vi "Threshold Obstacles.vi"(8 "error in (no error)":errorcluster, 10 "Threshold":dbl, 11 "Simulator in":refnum<class "Simulator.lvclass">) -> (0 "error out":errorcluster, 2 "Obstacles Within Threshold":cluster{"x":dbl, "y":dbl}[](array[cluster]), 3 "Simulator out":refnum<class "Simulator.lvclass">)   [LabVIEW 2011, in "Simulator.lvclass"]
uses:
  Simulator.lvclass
  Simulator.lvclass/Simulator.ctl
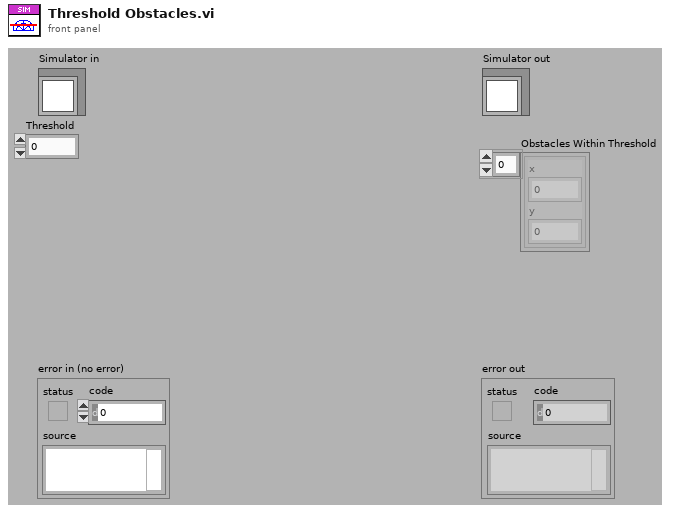
[diagram p1: front panel]
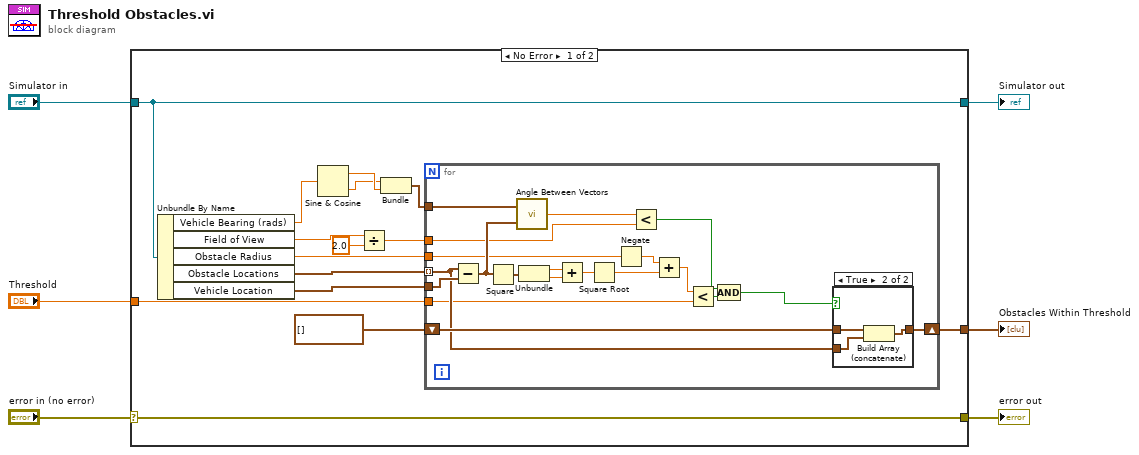
[diagram p0: block diagram]
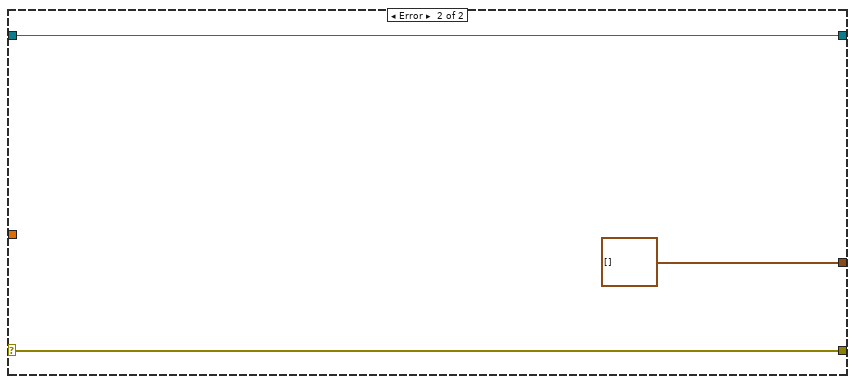
[diagram p3: hidden frame]
diagram:
  n1 = case shown="No Error" "error in (no error)" {
    selector: "error in (no error)" -> [w21 w48]
    tunnel: [w21 w48] -> w5
    tunnel: [w20 w47] -> w3
    tunnel: "Simulator in" -> [w20 w47]
    tunnel: "Threshold" -> [w16 _]
    tunnel: [w15 cluster{"x":dbl, "y":dbl}[] [] ("Obstacle Locations")] -> w1
    frame No Error {
      n2 = Unbundle By Name(w20) -> ("Vehicle Bearing (rads)"=w11:dbl, "Field of View"=w14:dbl, "Obstacle Radius"=w7:dbl, "Obstacle Locations"=w18:cluster{"x":dbl, "y":dbl}[], "Vehicle Location"=w19:cluster{"x":dbl, "y":dbl})
      n3 = Sine & Cosine(0:w11) -> (1:w9:dbl, 2:w8:dbl)
      n4 = Divide(x=w14, y=2.0) -> (x/y=w12:dbl)
      n5 = Bundle(w8, w9) -> (w10:cluster{dbl, dbl})  [unwired: 1 in]
      n6 = for {
        tunnel: w19 -> [w41]
        tunnel: w18 -> [w35] mode=indexing
        shift-right: [w34] -> w15
        shift-left: cluster{"x":dbl, "y":dbl}[] [] ("Obstacle Locations") -> [w36]
        tunnel: w16 -> [w33]
        tunnel: w12 -> [w29]
        tunnel: w10 -> [w27]
        tunnel: w7 -> [w24]
        n7 = Subtract(x=w35, y=w41) -> (x-y=w30:cluster{"x":dbl, "y":dbl})
        n8 = Square(x=w30) -> (x^2=w40:cluster{"x":dbl, "y":dbl})
        n9 = call "Angle Between Vectors.vi"("B"=w30, "A"=w27) -> ("Angle (rads)"=w28:dbl)
        n10 = Unbundle(w40) -> ("x"=w39:dbl, "y"=w38:dbl)
        n11 = Add(x=w39, y=w38) -> (x+y=w37:dbl)
        n12 = Square Root(x=w37) -> (sqrt(x)=w26:dbl)
        n13 = Negate(x=w24) -> (-x=w23:dbl)
        n14 = Less?(x=w28, y=w29) -> (x < y?=w22:bool)
        n15 = Add(x=w23, y=w26) -> (x+y=w25:dbl)
        n16 = Less?(x=w25, y=w33) -> (x < y?=w32:bool)
        n17 = Compound Arithmetic op=AND(w22, w32) -> (w31:bool)
        n18 = case shown="True" w31 {
          tunnel: w36 -> [w42 w45]
          tunnel: w35 -> [_ w44]
          tunnel: [w42 w43] -> w34
          frame False {
          }
          frame True {
            n19 = Build Array (concatenate)(w45, w44) -> (w43:cluster{"x":dbl, "y":dbl}[])
          }
        }
      }
    }
    frame Error {
    }
  }
  "error out" <- w5
  "Simulator out" <- w3
  "Obstacles Within Threshold" <- w1
